vi "GUI_HTT_MultiCamDriveAmpV4.vi"() -> ()   [LabVIEW 2020]
uses:
  Shared/GUI_Template/GUI_master/tcp_new_data_event.ctl
  Shared/GUI_Template/GUI_master/tcp new data cluster.ctl
  General GUIs/Device GUIs/GUI_Cameras/Controls/Crosshair type def.ctl
  <userlib>/_OpenG.lib/array/array.llb/Filter 1D Array with Scalar (String)__ogtk.vi
panel:
  out "Current State":string
  out "String 4":string="x1\ny1\nx2\ny2"
  out "String 3":string="x1\ny1\nx2\ny2"
  out "String 2":string="x1\ny1\nx2\ny2"
  out "String":string="x1\ny1\nx2\ny2"
  in  "visibility":bool=TRUE
  out "appended array":string[](array[string]) caption="XH"
  out "appended array 6":string[](array[string]) caption="XH"
  out "appended array 8":string[](array[string]) caption="XH"
  out "appended array 4":string[](array[string]) caption="XH"
  in  "UDP error message":string
  out "tcp data event 2":T1
  out "error IO 2":errorcluster
  in  "Color Box":u32(colorbox)
  in  "TargetSize.Y::5":dbl=45.0 caption="y" min=2.0 max=3000.0 format="%#_6f"
  in  "TargetSize.X::5":dbl=47.0 caption="x" min=2.0 max=3000.0 format="%#_6f"
  in  "TargetSize.Y::4":dbl=45.0 caption="y" min=2.0 max=3000.0 format="%#_6f"
  in  "TargetSize.X::4":dbl=47.0 caption="x" min=2.0 max=3000.0 format="%#_6f"
  in  "TargetSize.Y::3":dbl=163.0 caption="y" min=2.0 max=3000.0 format="%#_6f"
  in  "TargetSize.X::3":dbl=152.0 caption="x" min=2.0 max=3000.0 format="%#_6f"
  in  "TargetSize.Y::2":dbl=74.0 caption="y" min=2.0 max=3000.0 format="%#_6f"
  in  "TargetSize.X::2":dbl=75.0 caption="x" min=2.0 max=3000.0 format="%#_6f"
  in  "active cams":string
  out "CCDs":string[](array[string])
  out "Cameras":T2
  in  "Target.Y::5":dbl=45.0 caption="y" min=0.0 max=2000.0 format="%#_6f"
  in  "Target.X::5":dbl=47.0 caption="x" min=0.0 max=2000.0 format="%#_6f"
  in  "Target.Y::4":dbl=45.0 caption="y" min=0.0 max=2000.0 format="%#_6f"
  in  "Target.X::4":dbl=47.0 caption="x" min=0.0 max=2000.0 format="%#_6f"
  in  "Target.Y::3":dbl=163.0 caption="y" min=0.0 max=2000.0 format="%#_6f"
  in  "Target.X::3":dbl=152.0 caption="x" min=0.0 max=2000.0 format="%#_6f"
  in  "Target.Y::2":dbl=74.0 caption="y" min=0.0 max=2000.0 format="%#_6f"
  in  "Target.X::2":dbl=75.0 caption="x" min=0.0 max=2000.0 format="%#_6f"
  out "error out":errorcluster
  in  "triggerdelay::5":dbl=0.001 caption="triggerdelay" min=0.0 max=1000000.0 format="%_4p"
  in  "triggerdelay::4":dbl=0.001 caption="triggerdelay" min=0.0 max=1000000.0 format="%_4p"
  in  "triggerdelay::3":dbl=0.001 caption="triggerdelay" min=0.0 max=100000.0 format="%_4p"
  in  "triggerdelay::2":dbl=0.001 caption="triggerdelay" min=0.0 max=1000000.0 format="%_4p"
  in  "trigger::5":bool caption="Trigger"
  in  "centroidy::5":dbl=0.001 caption="centroid y" min=0.0 max=0.0 format="%_4f"
  in  "centroidx::5":dbl=0.001 caption="centroid x" min=0.0 max=0.0 format="%_4f"
  in  "exposure::5":dbl=0.001 caption="exposure" min=9e-05 max=1.0 format="%_4p"
  out "image::5":T3(plugin-control) caption="HTT-MagCam-01"
  in  "GUIdevice 5":string="HTT-D-AMP4_Out"
  in  "trigger::4":bool caption="Trigger"
  in  "centroidy::4":dbl=0.001 caption="centroid y" min=0.0 max=0.0 format="%_4f"
  in  "centroidx::4":dbl=0.001 caption="centroid x" min=0.0 max=0.0 format="%_4f"
  in  "exposure::4":dbl=0.001 caption="exposure" min=9e-05 max=10.0 format="%_4p"
  out "image::4":T3(plugin-control) caption="HTT-MagCam-02"
  in  "GUIdevice 4":string="HTT-D-AMP4_In"
  in  "trigger::3":bool caption="Trigger"
  in  "centroidy::3":dbl=0.001 caption="centroid y" min=0.0 max=0.0 format="%_4f"
  in  "centroidx::3":dbl=0.001 caption="centroid x" min=0.0 max=0.0 format="%_4f"
  in  "exposure::3":dbl=0.001 caption="exposure" min=9e-05 max=10.0 format="%_4p"
  out "image::3":T3(plugin-control) caption="HTT-MagCam-03"
  in  "GUIdevice 3":string="HTT-D-AMP3_In"
  in  "trigger::2":bool caption="Trigger"
  in  "centroidy::2":dbl=0.001 caption="centroid y" min=0.0 max=0.0 format="%_4f"
  in  "centroidx::2":dbl=0.001 caption="centroid x" min=0.0 max=0.0 format="%_4f"
  in  "exposure::2":dbl=0.001 caption="exposure" min=9e-05 max=10.0 format="%_4p"
  out "image::2":T3(plugin-control) caption="HTT-MagCam-04"
  in  "GUIdevice 2":string="HTT-D-AMP2_In"
  out "tcp data event":T1
  in  "Refresh Button":bool caption="Update Crosshairs"
  in  "Select device":string(combo)="FrogHPD"
  in  "stop":bool
  in  "GUIdevice 1":string="HPD_CCD"
  out "image1 4":T3(plugin-control)
  out "image1 3":T3(plugin-control)
  out "image1 2":T3(plugin-control)
  out "image1":T3(plugin-control)
  # "XHair location"
  # "XHair location"
  # "XHair size"
  # "XHair size"
  # "XHair location"
  # "XHair size"
  # "XHair size"
  # "XHair location"
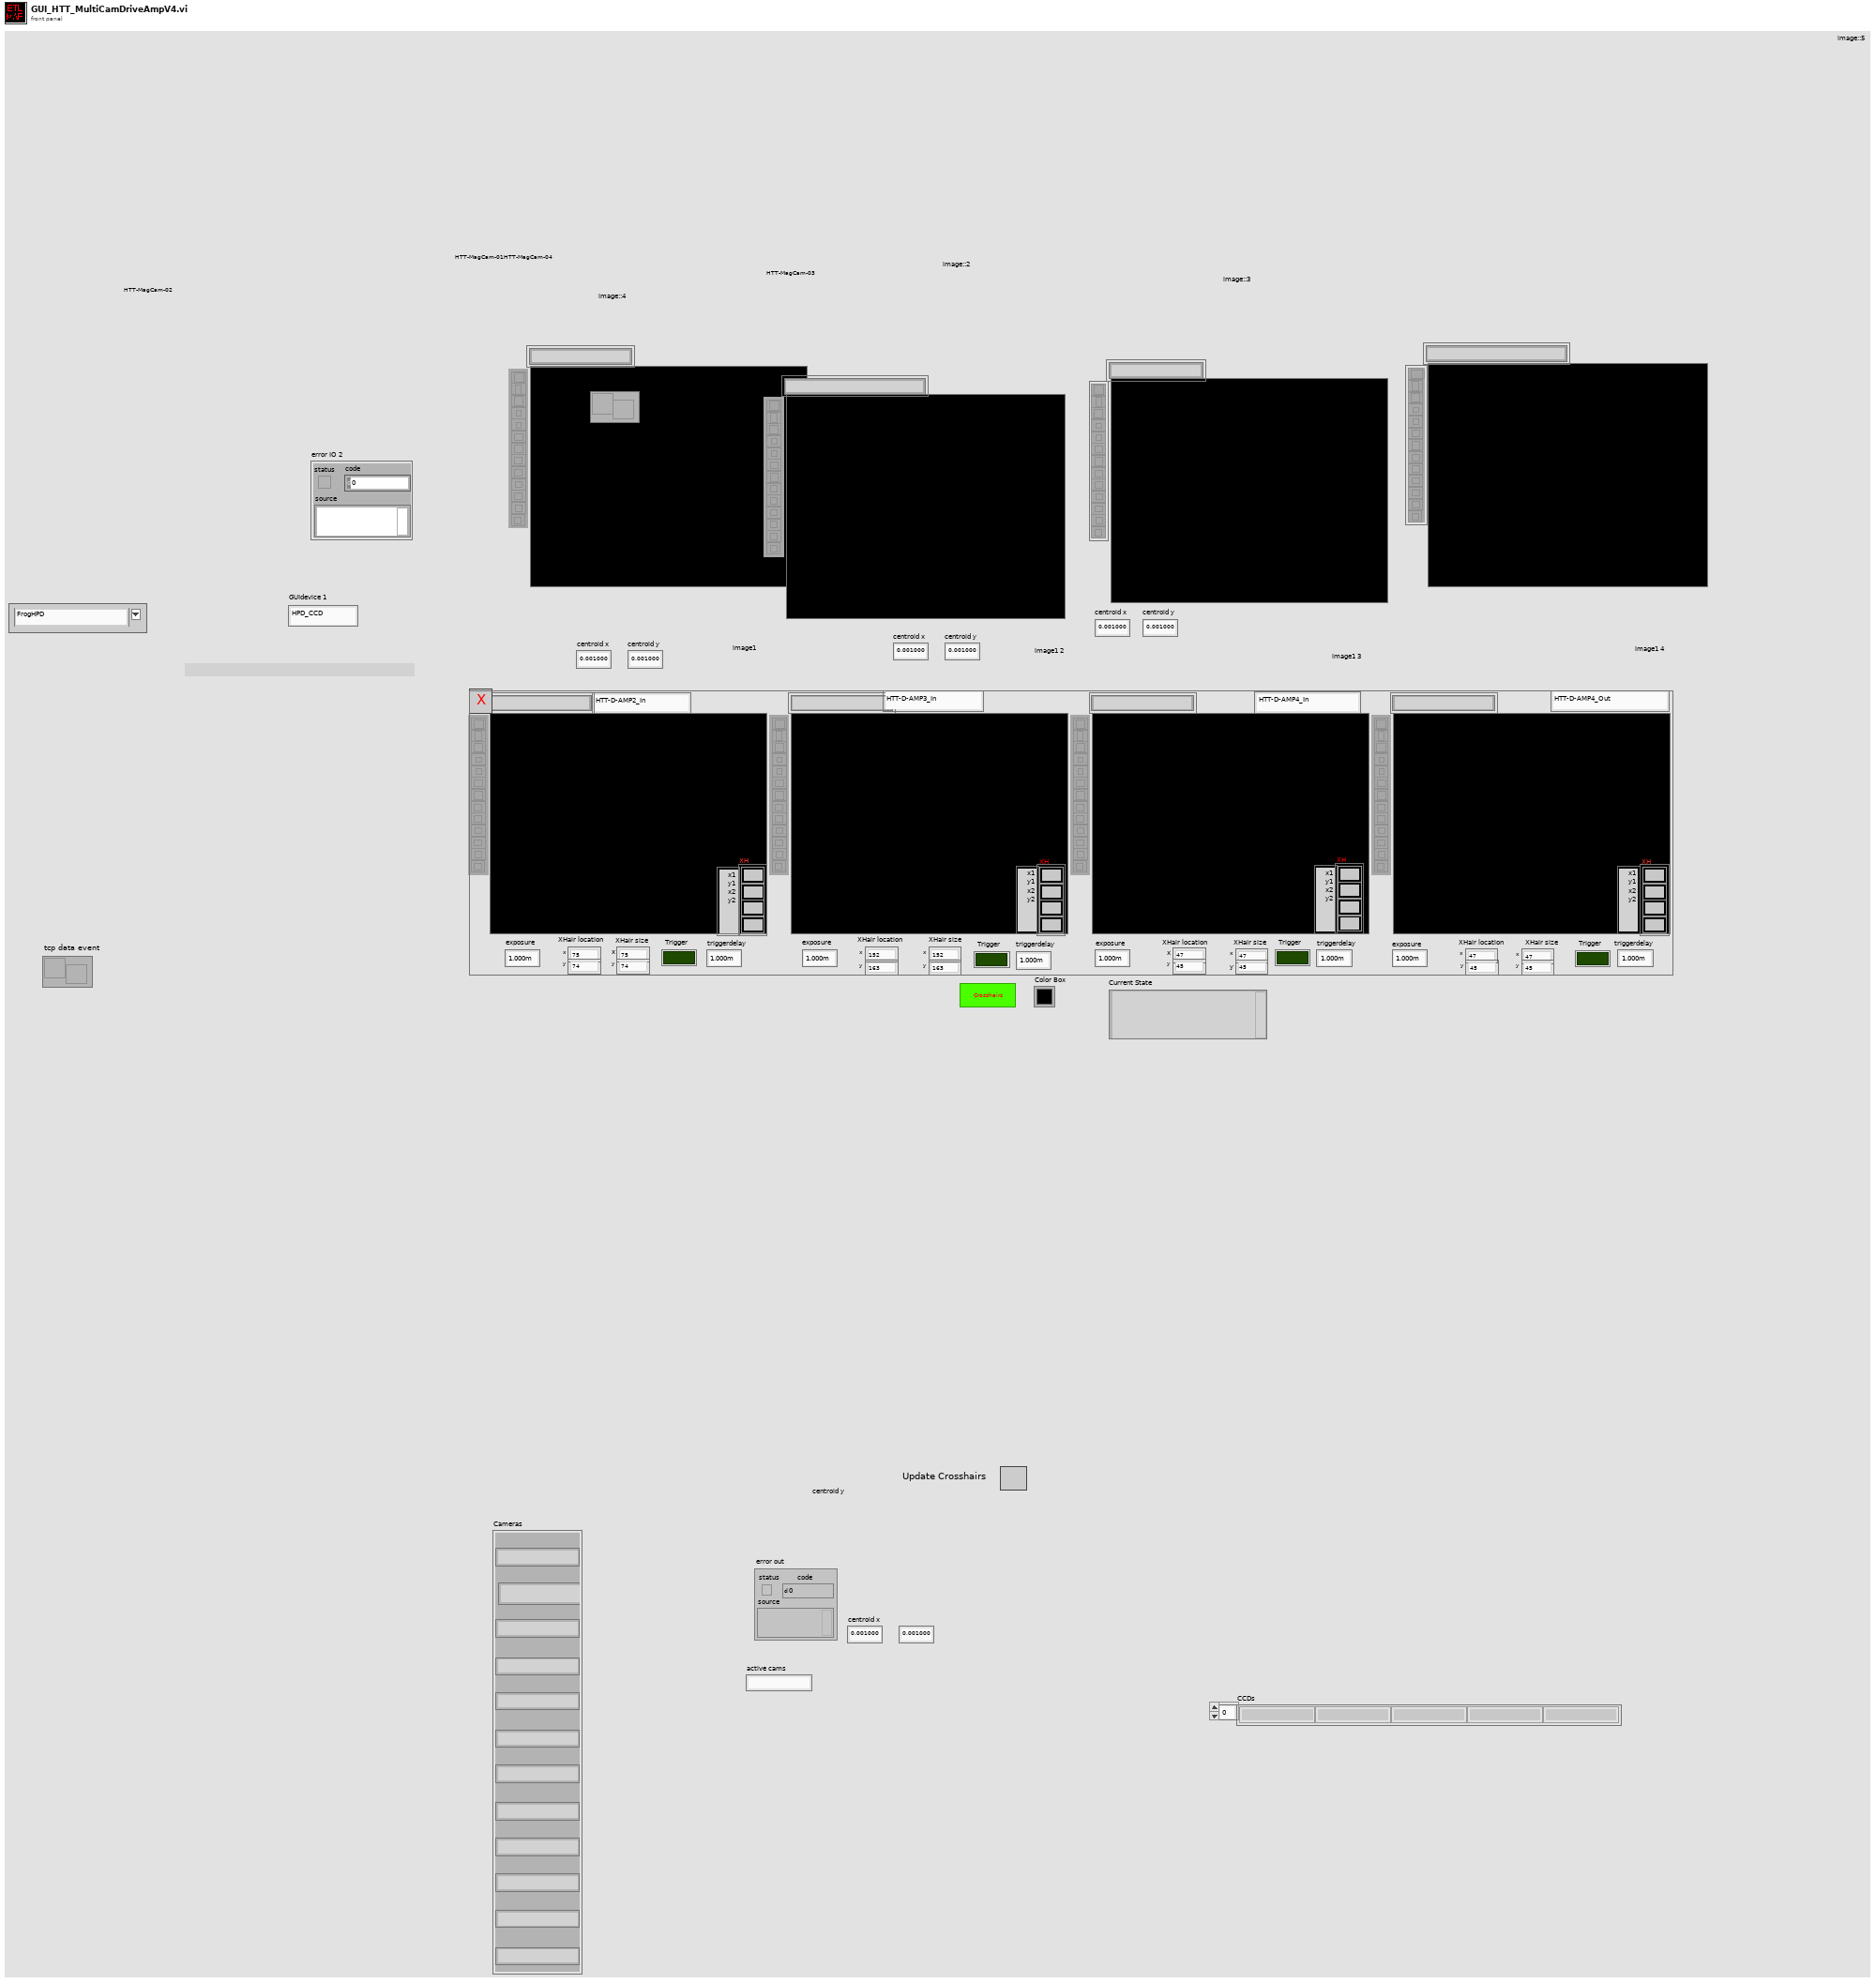
[diagram p1: front panel]
types:
  T1 = typedef "tcp_new_data_event.ctl" = refnum<user-event>
  T2 = cluster{"[0]":string, "[1]":string, "[2]":string, "[3]":string, "[4]":string, "[5]":string, "[6]":string, "[7]":string, "[8]":string, "[8] 2":string, "[8] 3":string, "[8] 4":string}
  T3 = typedef "IMAQ Image.ctl" = refnum<image>
  T4 = typedef "Image Type" = u32
  T5 = cluster{"Target.X::2":refnum<vi>, "Target.Y::2":refnum<vi>}
  T6 = cluster{"Target.X::3":refnum<vi>, "Target.Y::3":refnum<vi>}
  T7 = cluster{"Target.X::4":refnum<vi>, "Target.Y::4":refnum<vi>}
  T8 = cluster{"Target.X::5":refnum<vi>, "Target.Y::5":refnum<vi>}
  T9 = cluster{"TargetSize.X::2":refnum<vi>, "TargetSize.Y::2":refnum<vi>}
  T10 = cluster{"TargetSize.X::3":refnum<vi>, "TargetSize.Y::3":refnum<vi>}
  T11 = cluster{"TargetSize.X::4":refnum<vi>, "TargetSize.Y::4":refnum<vi>}
  T12 = cluster{"TargetSize.X::5":refnum<vi>, "TargetSize.Y::5":refnum<vi>}
  T13 = cluster{"Target.X::5":refnum<vi>, "Target.Y::5":refnum<vi>}[]
  T14 = cluster{"TargetSize.X::5":refnum<vi>, "TargetSize.Y::5":refnum<vi>}[]
  T15 = cluster{"[0]":string, "[1]":string, "[2]":string, "[3]":string, "[4]":string, "[5]":string, "[6]":string, "[7]":string, "[8]":string, "[9]":string, "[10]":string, "[11]":string}
  T16 = typedef "Crosshair type def.ctl" = cluster{"Draw":bool, "Target":cluster{"x":dbl, "y":dbl}, "Size":cluster{"x":dbl, "y":dbl}, "Angle":dbl, "Color":u32, "Thickness":u8, "CrosshairLabel":string}
  T17 = cluster{"Left":i32, "Top":i32, "Right":i32, "Bottom":i32}
  T18 = enum32{"invalid app kind", "Development System", "Run Time System", "Student Edition", "Embedded LabVIEW", "Evaluation", "Custom"}
  T19 = typedef "tcp new data cluster.ctl" = cluster{"EventEnum":enum16{"new data", "connection status update"}, "Device name":string}
  T20 = enum32{"Invalid", "Standard", "Closed", "Hidden", "Minimized", "Maximized"}
  T21 = cluster{"Core":cluster{"Current VI Reference":refnum<vi>, "Close Panel on Exit?":bool}, "Your Boolean data":bool, "active cams":string, "SuperGUI":cluster{"STOP queue":refnum<queue>, "SuperGUI ref":refnum<vi>}}
  T22 = cluster{"STOP queue":refnum<queue>, "SuperGUI ref":refnum<vi>}
  T23 = cluster{"Current VI Reference":refnum<vi>, "Close Panel on Exit?":bool}
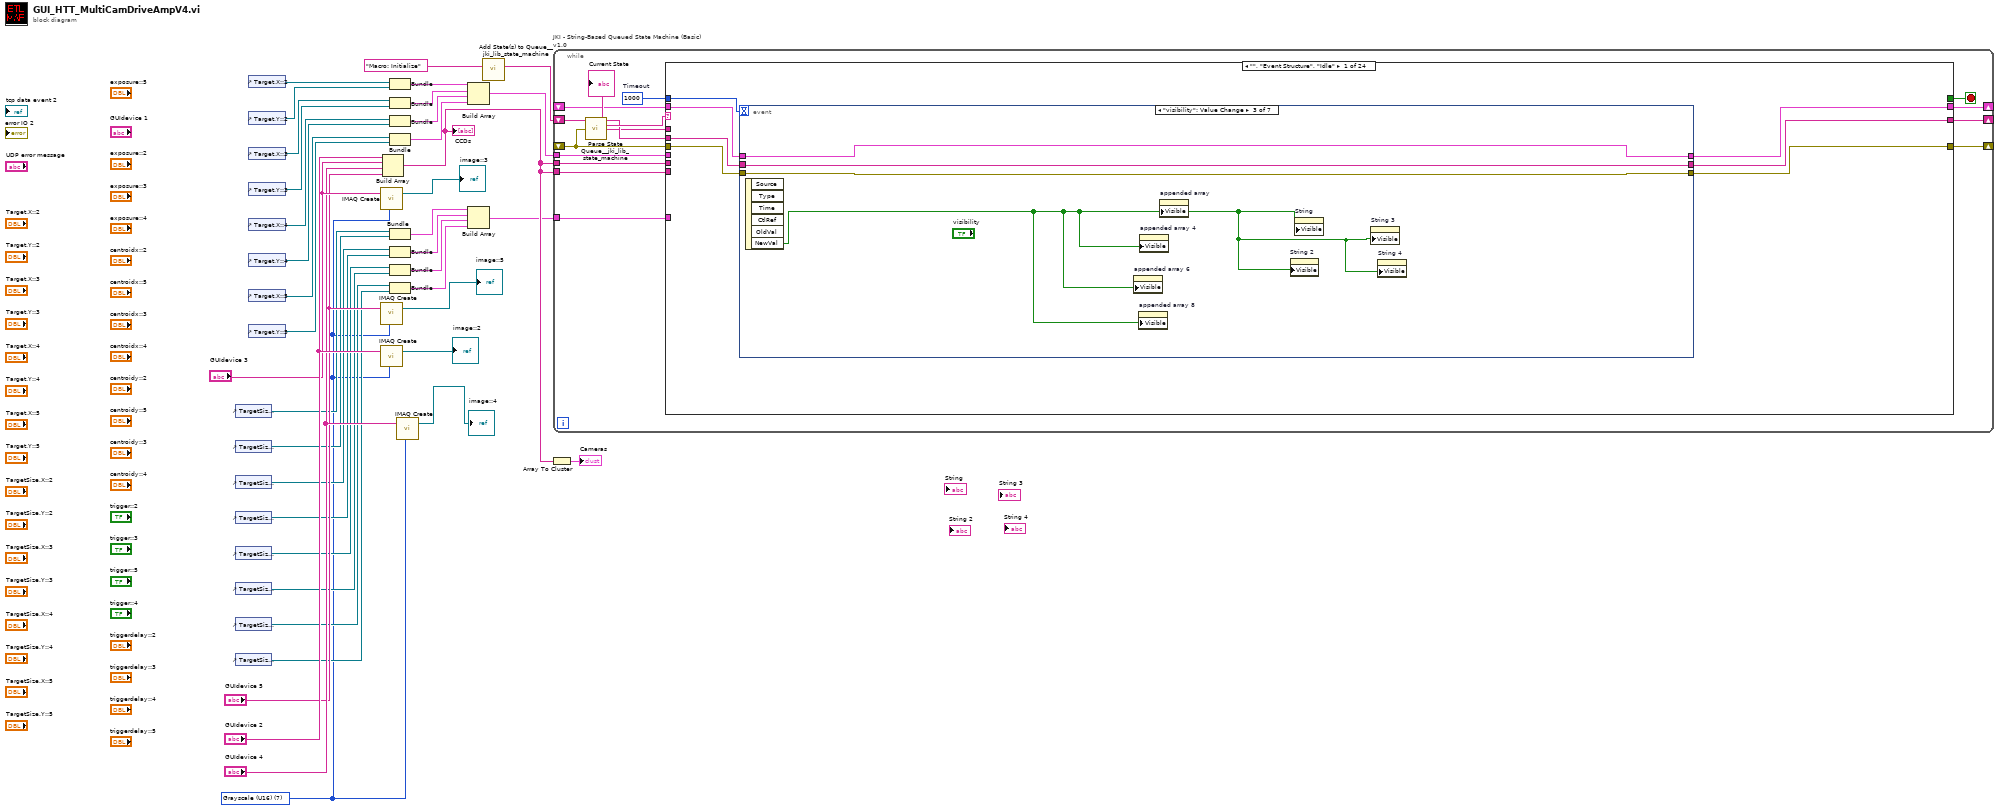
[diagram p0: block diagram]
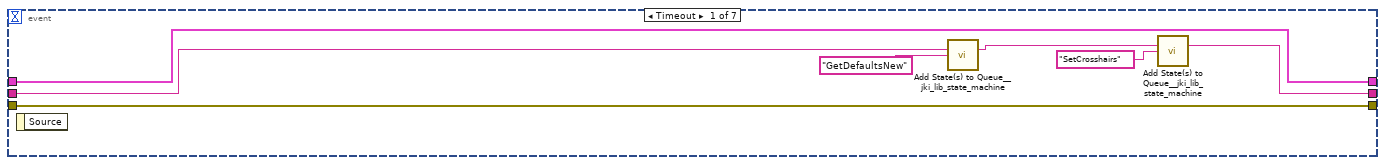
[diagram p2: hidden frame]
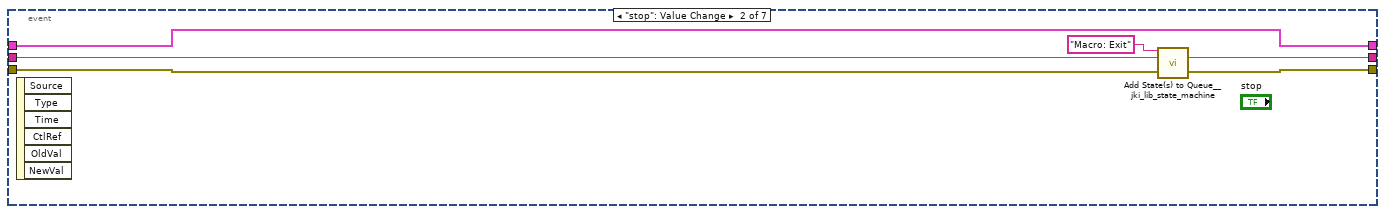
[diagram p3: hidden frame]
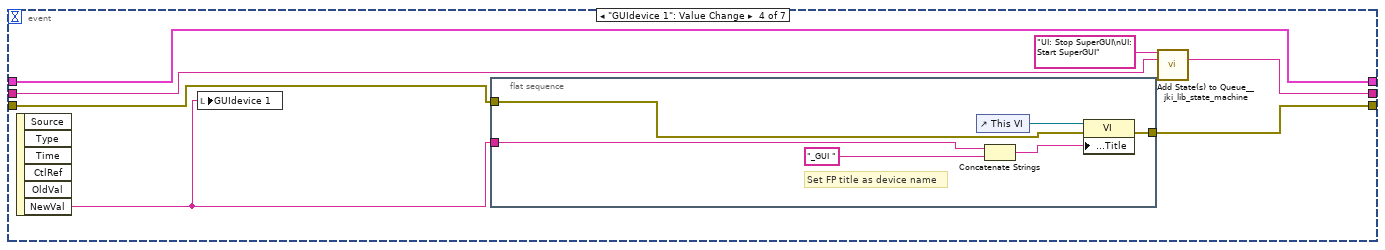
[diagram p4: hidden frame]
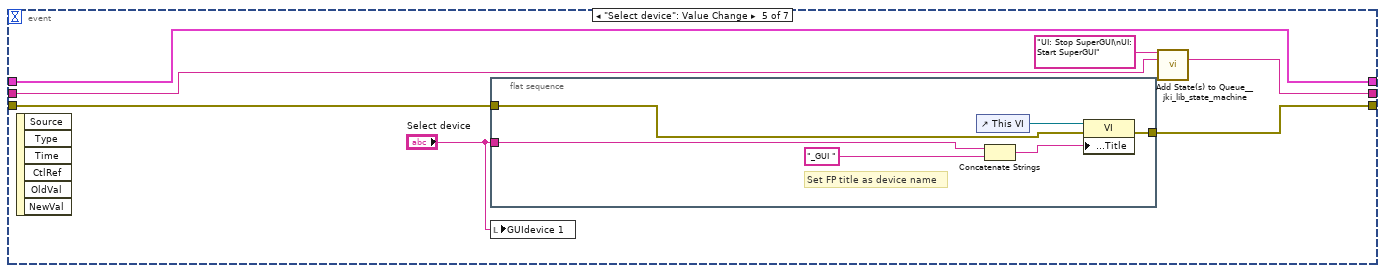
[diagram p5: hidden frame]
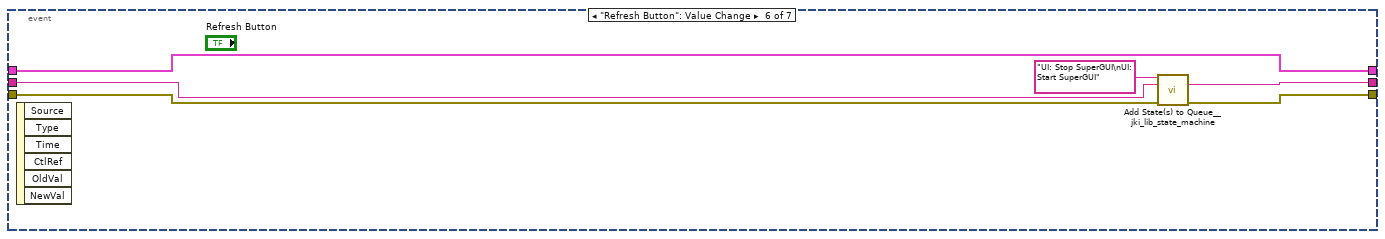
[diagram p6: hidden frame]
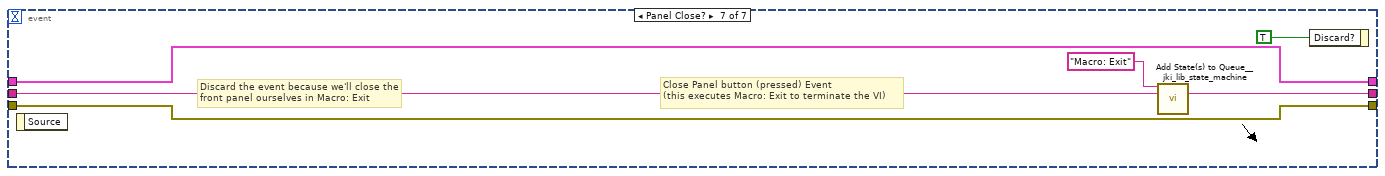
[diagram p7: hidden frame]
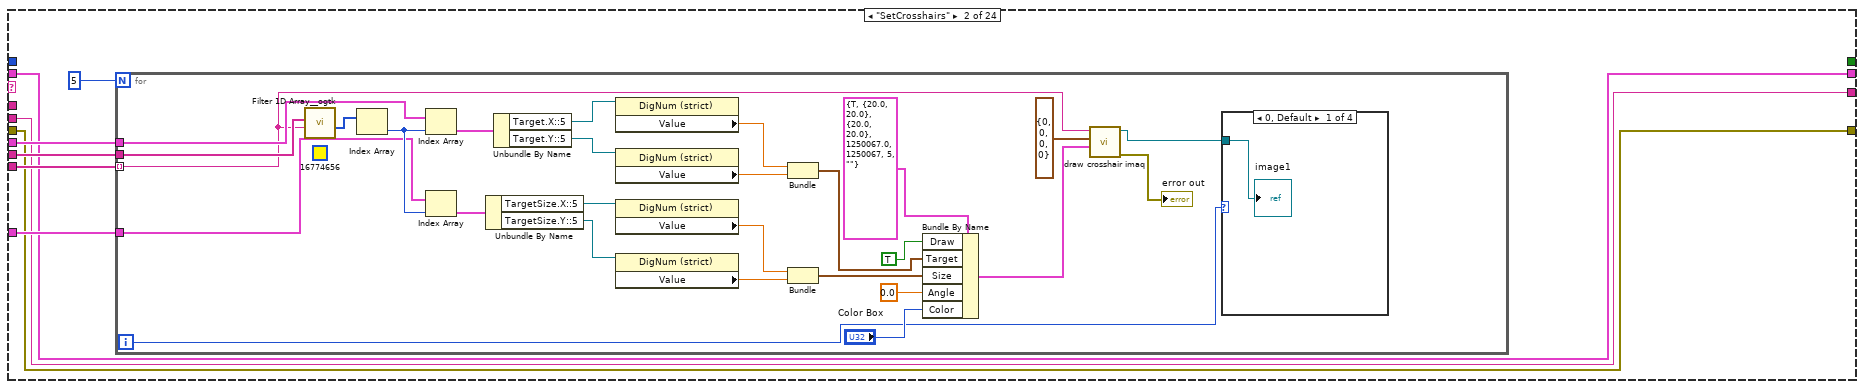
[diagram p8: hidden frame]
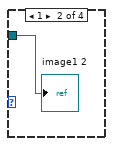
[diagram p9: hidden frame]
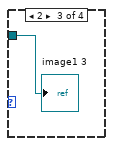
[diagram p10: hidden frame]
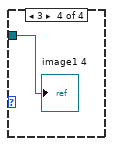
[diagram p11: hidden frame]
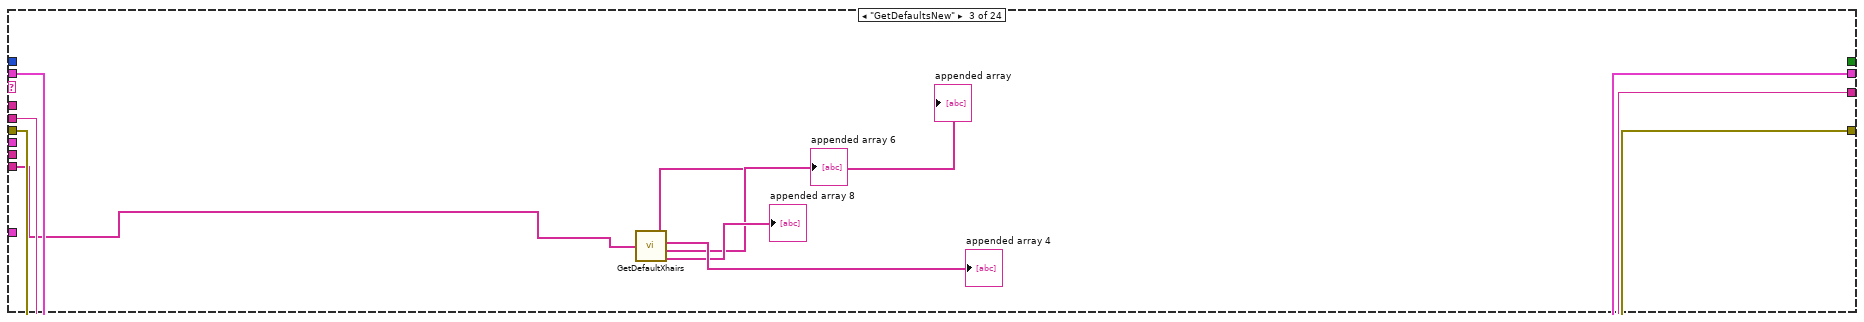
[diagram p12: hidden frame]
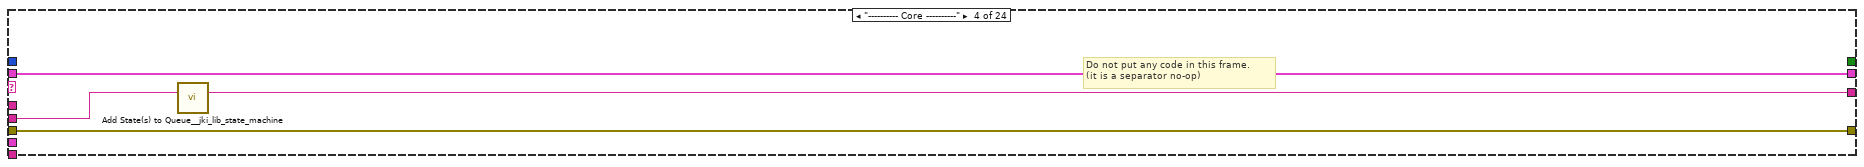
[diagram p13: hidden frame]
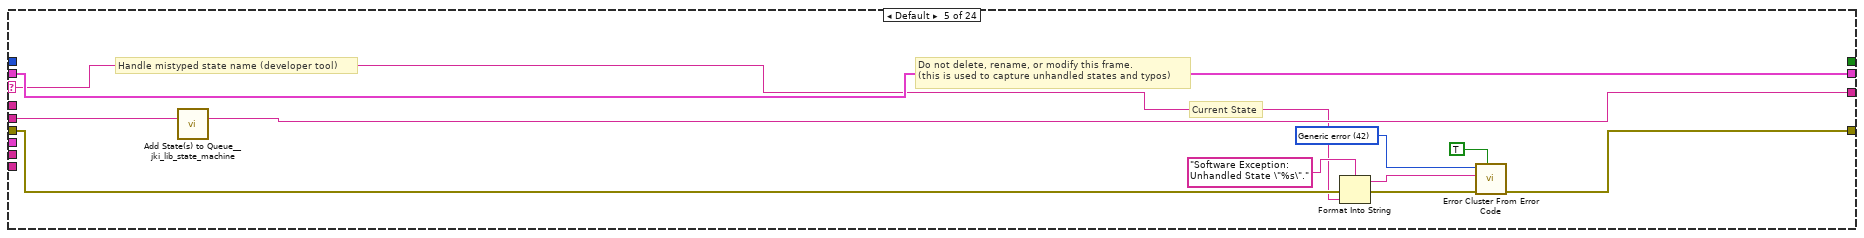
[diagram p14: hidden frame]
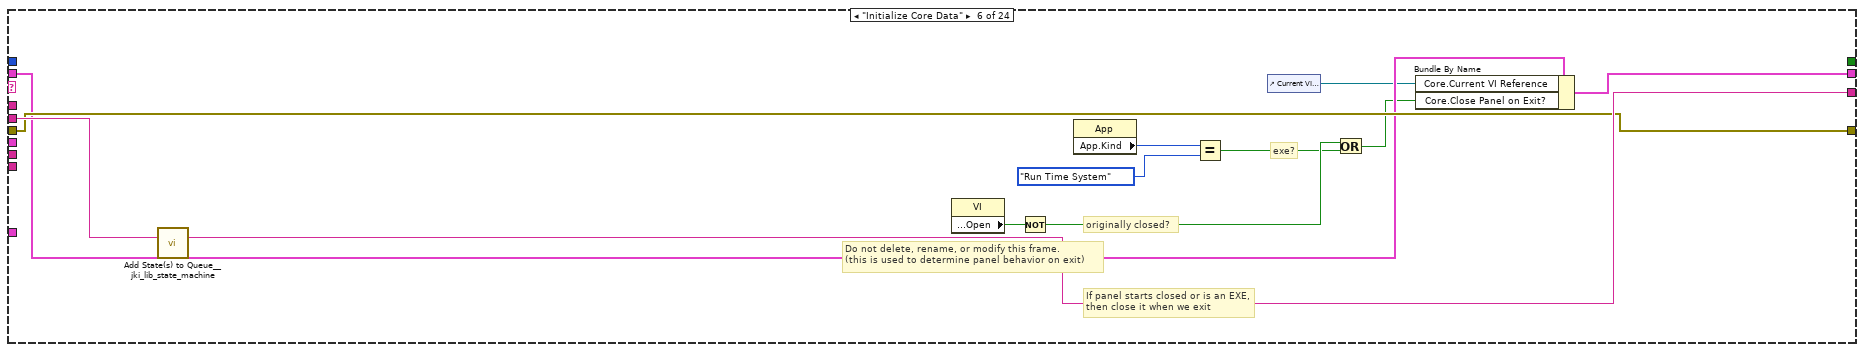
[diagram p15: hidden frame]
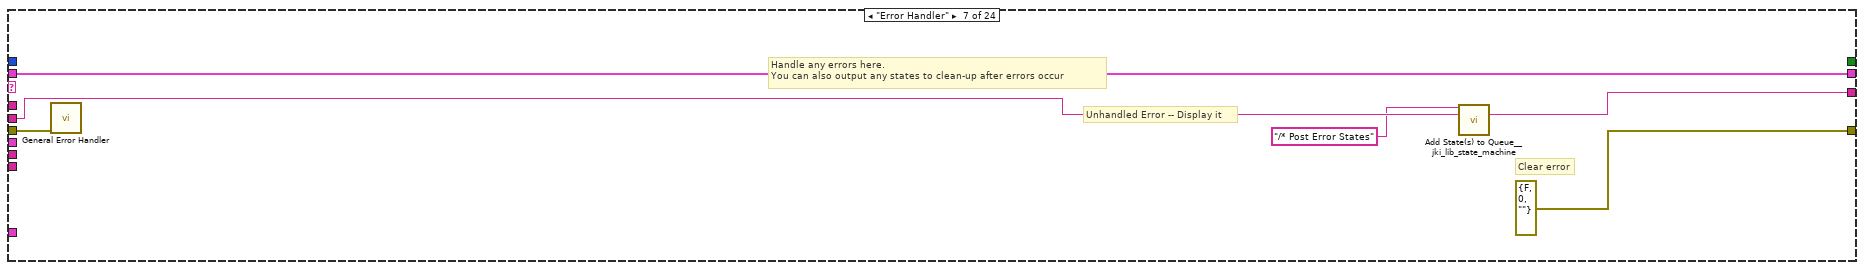
[diagram p16: hidden frame]
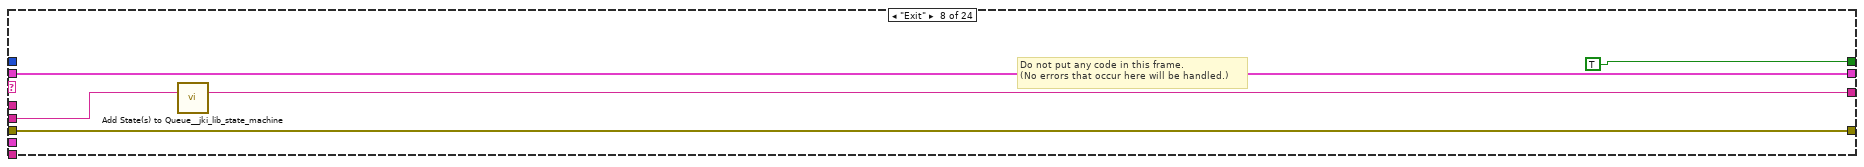
[diagram p17: hidden frame]
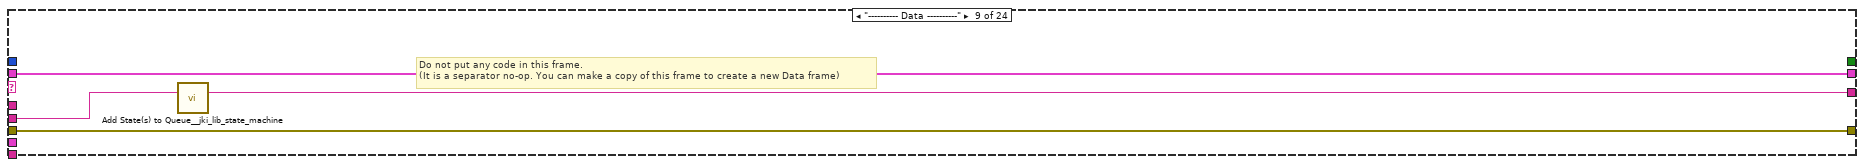
[diagram p18: hidden frame]
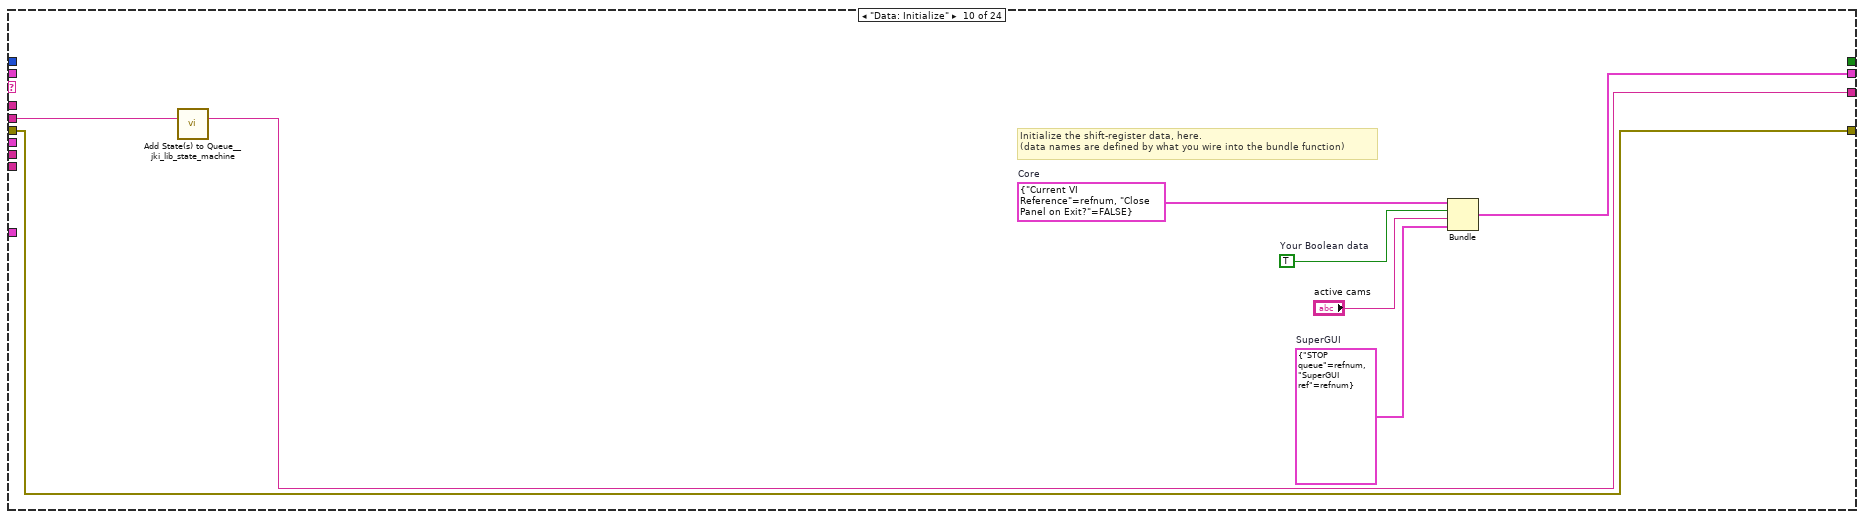
[diagram p19: hidden frame]
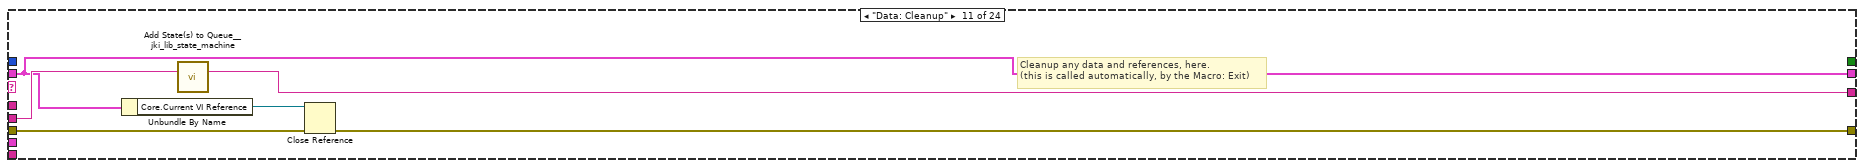
[diagram p20: hidden frame]
diagram:
  w2 = T4 7 items=["Grayscale (U8)", "Grayscale (I16)", "Grayscale (SGL)", "Complex (CSG)", "RGB (U32)", "HSL (U32)", "RGB (U64)", "Grayscale (U16)"] ("Image Type")
  n1 = control-ref of="TargetSize.X::2"() -> (w15:refnum<vi>)
  n2 = control-ref of="TargetSize.Y::2"() -> (w14:refnum<vi>)
  n3 = control-ref of="TargetSize.X::3"() -> (w13:refnum<vi>)
  n4 = control-ref of="TargetSize.Y::3"() -> (w12:refnum<vi>)
  n5 = control-ref of="TargetSize.X::4"() -> (w11:refnum<vi>)
  n6 = control-ref of="TargetSize.Y::4"() -> (w10:refnum<vi>)
  n7 = control-ref of="TargetSize.X::5"() -> (w9:refnum<vi>)
  n8 = control-ref of="TargetSize.Y::5"() -> (w8:refnum<vi>)
  n9 = control-ref of="Target.X::2"() -> (w34:refnum<vi>)
  n10 = control-ref of="Target.Y::2"() -> (w33:refnum<vi>)
  n11 = control-ref of="Target.X::3"() -> (w32:refnum<vi>)
  n12 = control-ref of="Target.Y::3"() -> (w31:refnum<vi>)
  n13 = control-ref of="Target.X::4"() -> (w30:refnum<vi>)
  n14 = control-ref of="Target.Y::4"() -> (w29:refnum<vi>)
  n15 = control-ref of="Target.X::5"() -> (w28:refnum<vi>)
  n16 = control-ref of="Target.Y::5"() -> (w27:refnum<vi>)
  n17 = call "IMAQ Create"("Image Name"="GUIdevice 3", "Image Type"=w2) -> ("New Image"=→"image::3":T3)  [unwired: 3 in, 1 out]
  n18 = call "IMAQ Create"("Image Name"="GUIdevice 5", "Image Type"=w2) -> ("New Image"=→"image::5":T3)  [unwired: 3 in, 1 out]
  n19 = call "IMAQ Create"("Image Name"="GUIdevice 2", "Image Type"=w2) -> ("New Image"=→"image::2":T3)  [unwired: 3 in, 1 out]
  n20 = Build Array("GUIdevice 2", "GUIdevice 3", "GUIdevice 4", "GUIdevice 5") -> (w16:string[])
  "CCDs" <- w16
  n21 = Bundle("Target.X::2"=w34, "Target.Y::2"=w33) -> (w26:T5)  [unwired: 1 in]
  n22 = Bundle("Target.X::3"=w32, "Target.Y::3"=w31) -> (w25:T6)  [unwired: 1 in]
  n23 = Bundle("Target.X::4"=w30, "Target.Y::4"=w29) -> (w23:T7)  [unwired: 1 in]
  n24 = Bundle("Target.X::5"=w28, "Target.Y::5"=w27) -> (w24:T8)  [unwired: 1 in]
  n25 = Bundle("TargetSize.X::2"=w15, "TargetSize.Y::2"=w14) -> (w7:T9)  [unwired: 1 in]
  n26 = Bundle("TargetSize.X::3"=w13, "TargetSize.Y::3"=w12) -> (w6:T10)  [unwired: 1 in]
  n27 = Bundle("TargetSize.X::4"=w11, "TargetSize.Y::4"=w10) -> (w4:T11)  [unwired: 1 in]
  n28 = Bundle("TargetSize.X::5"=w9, "TargetSize.Y::5"=w8) -> (w5:T12)  [unwired: 1 in]
  n29 = call "IMAQ Create"("Image Name"="GUIdevice 4", "Image Type"=w2) -> ("New Image"=→"image::4":T3)  [unwired: 3 in, 1 out]
  n30 = Build Array(w26, w25, w23, w24) -> (w22:T13)
  n31 = Build Array(w7, w6, w4, w5) -> (w3:T14)
  n32 = call <vilib>:"Add State(s) to Queue__jki_lib_state_machine.vi"("State(s) in (\"\")"="Macro: Initialize") -> ("States Out"=w39:string)  [unwired: 14 in]
  n33 = Array To Cluster(array=w16) -> (cluster=→"Cameras":T15)
  n34 = while "JKI - String-Based Queued State Machine (Basic) v1.0" {
    shift-right: [w47] -> _
    shift-left: _ -> [w44]
    shift-right: [w50] -> _
    shift-left: _ -> [w45]
    shift-right: [w49] -> _
    shift-left: w39 -> [w51]
    tunnel: w22 -> [w41]
    tunnel: w16 -> [w42]
    tunnel: w16 -> [w43]
    tunnel: w3 -> [w40]
    stop <- w48 stop-if-true
    w46 = 1000  # Timeout
    n35 = call <vilib>:"Parse State Queue__jki_lib_state_machine.vi"("State Queue"=w51, "Error In (no error)"=w45) -> ("Remaining States"=w53:string, "Current State"=w54:string, "Arguments"=w52:string)  [unwired: 11 in]
    "Current State" <- w54
    n36 = case shown="\"\", \"Event Structure\", \"Idle\"" w54 {
      selector: w54 -> [_ _ _ _ w166 _ _ _ _ _ _ _ _ _ _ _ _ _ _ _ _ _ _ _]
      tunnel: w53 -> [w61 w117 w160 w165 w170 w188 w194 w199 w203 w211 w217 w221 w226 w232 w267 w275 w281 w292 w318 w323 w334 w338 w342 w346]
      tunnel: w52 -> [_ _ _ _ _ _ _ _ _ _ _ _ _ _ _ _ w276 w286 _ _ _ _ _ _]
      tunnel: w44 -> [w59 w118 w161 w162 w168 w179 w191 w197 w200 _ w212 w218 w224 w230 w258 w270 w279 w288 w315 w320 w331 w335 w339 w343]
      tunnel: [w58 w116 w159 w163 w172 w185 errorcluster {"status"=FALSE, "code"=0, "source"=""} ("error out") w196 w201 w208 w213 w219 w222 w227 w251 w268 w277 w289 w316 w321 w332 w336 w340 w344] -> w50
      tunnel: w45 -> [w57 w116 w159 w163 w171 w185 w190 w196 w201 w208 w214 w219 w223 w228 w252 w269 w278 w290 w316 w321 w332 w336 w340 w344]
      tunnel: [w60 w117 w160 w164 w169 w187 w193 w198 w202 w210 w216 w220 w225 w231 w266 w274 w280 w291 w317 w322 w333 w337 w341 w345] -> w49
      tunnel: [_ _ _ _ _ _ _ TRUE _ _ _ _ _ _ _ _ _ _ _ _ _ _ _ _] -> w48
      tunnel: [w56 w118 w161 w162 w168 w186 w191 w197 w200 w209 w212 w218 w224 w230 w257 w270 w279 w288 w315 w320 w331 w335 w339 w343] -> w47
      tunnel: w46 -> [w55 _ _ _ _ _ _ _ _ _ _ _ _ _ _ _ _ _ _ _ _ _ _ _]
      tunnel: w43 -> [_ w120 w158 _ _ _ _ _ _ _ _ _ _ _ _ _ _ _ _ _ _ _ _ _]
      tunnel: w42 -> [_ w121 _ _ _ _ _ _ _ _ _ _ _ _ _ _ _ _ _ _ _ _ _ _]
      tunnel: w41 -> [_ w122 _ _ _ _ _ _ _ _ _ _ _ _ _ _ _ _ _ _ _ _ _ _]
      tunnel: w40 -> [_ w119 _ _ _ _ _ _ _ _ _ _ _ _ _ _ _ _ _ _ _ _ _ _]
      frame "", "Event Structure", "Idle" {
        n37 = event shown="[2] \"visibility\": Value Change" {
          selector: _ -> [_ _ _ _ _ _ _]
          dyn-events: _ -> [_ _ _ _ _ _ _]
          timeout: w55 -> [_ _ _ _ _ _ _]
          tunnel: w61 -> [w64 w71 w75 w81 w93 w106 w114]
          tunnel: [w68 w70 w75 w80 w92 w105 w113] -> w60
          tunnel: w59 -> [w66 w73 w77 w84 w97 w108 w111]
          tunnel: [w67 w72 w76 w82 w95 w107 w112] -> w58
          tunnel: w57 -> [w67 w72 w76 w83 w96 w107 w112]
          tunnel: [w66 w73 w77 w84 w97 w108 w111] -> w56
          event Timeout {
            n38 = event-data() -> ()  [unwired: 1 in, 1 out]
            n39 = call <vilib>:"Add State(s) to Queue__jki_lib_state_machine.vi"("State(s) in (\"\")"=w64, "State(s) at Back (\"\")"="GetDefaultsNew") -> ("States Out"=w62:string)  [unwired: 13 in]
            n40 = call <vilib>:"Add State(s) to Queue__jki_lib_state_machine.vi"("State(s) in (\"\")"=w62, "State(s) at Back (\"\")"="SetCrosshairs") -> ("States Out"=w68:string)  [unwired: 13 in]
          }
          event "stop": Value Change {
            n41 = event-data() -> ()  [unwired: 1 in, 6 out]
            n42 = call <vilib>:"Add State(s) to Queue__jki_lib_state_machine.vi"("State(s) in Front (\"\")"="Macro: Exit", "State(s) in (\"\")"=w71) -> ("States Out"=w70:string)  [unwired: 13 in]
          }
          event "visibility": Value Change {
            n43 = event-data() -> ("NewVal"=w74:bool)  [unwired: 1 in, 5 out]
            n44 = property on="appended array 6" class="Arr (strict)"("Visible"=w74) -> ()  [unwired: 2 in, 2 out]
            n45 = property on="appended array 8" class="Arr (strict)"("Visible"=w74) -> ()  [unwired: 2 in, 2 out]
            n46 = property on="appended array 4" class="Arr (strict)"("Visible"=w74) -> ()  [unwired: 2 in, 2 out]
            n47 = property on="appended array" class="Arr (strict)"("Visible"=w74) -> ()  [unwired: 2 in, 2 out]
            n48 = property on="String 2" class="Str"("Visible"=w74) -> ()  [unwired: 2 in, 2 out]
            n49 = property on="String" class="Str"("Visible"=w74) -> ()  [unwired: 2 in, 2 out]
            n50 = property on="String 3" class="Str"("Visible"=w74) -> ()  [unwired: 2 in, 2 out]
            n51 = property on="String 4" class="Str"("Visible"=w74) -> ()  [unwired: 2 in, 2 out]
          }
          event "GUIdevice 1": Value Change {
            n52 = event-data() -> ("NewVal"=w78:string)  [unwired: 1 in, 5 out]
            n53 = local write "GUIdevice 1"(w78) -> ()
            n54 = flat-sequence {
              tunnel: [w87] -> w82
              tunnel: w83 -> [w86]
              tunnel: w78 -> [w85]
              frame #0 {
                # "Set FP title as device name"
                n55 = control-ref of="This VI"() -> (w90:refnum<vi>)
                n56 = Concatenate Strings(w85, "_GUI ") -> (w89:string)
                n57 = property class="VI"(reference=w90, error in=w86, "Front Panel.Title"=w89) -> (error out=w87:errorcluster)  [unwired: 1 out]
              }
            }
            n58 = call <vilib>:"Add State(s) to Queue__jki_lib_state_machine.vi"("State(s) in Front (\"\")"="UI: Stop SuperGUI\nUI: Start SuperGUI", "State(s) in (\"\")"=w81) -> ("States Out"=w80:string)  [unwired: 13 in]
          }
          event "Select device": Value Change {
            n59 = event-data() -> ()  [unwired: 1 in, 6 out]
            n60 = flat-sequence {
              tunnel: [w100] -> w95
              tunnel: w96 -> [w99]
              tunnel: "Select device" -> [w98]
              frame #0 {
                # "Set FP title as device name"
                n61 = control-ref of="This VI"() -> (w103:refnum<vi>)
                n62 = Concatenate Strings(w98, "_GUI ") -> (w102:string)
                n63 = property class="VI"(reference=w103, error in=w99, "Front Panel.Title"=w102) -> (error out=w100:errorcluster)  [unwired: 1 out]
              }
            }
            n64 = local write "GUIdevice 1"("Select device") -> ()
            n65 = call <vilib>:"Add State(s) to Queue__jki_lib_state_machine.vi"("State(s) in Front (\"\")"="UI: Stop SuperGUI\nUI: Start SuperGUI", "State(s) in (\"\")"=w93) -> ("States Out"=w92:string)  [unwired: 13 in]
          }
          event "Refresh Button": Value Change {
            n66 = event-data() -> ()  [unwired: 1 in, 6 out]
            n67 = call <vilib>:"Add State(s) to Queue__jki_lib_state_machine.vi"("State(s) in Front (\"\")"="UI: Stop SuperGUI\nUI: Start SuperGUI", "State(s) in (\"\")"=w106) -> ("States Out"=w105:string)  [unwired: 13 in]
          }
          event Panel Close? {
            # "Discard the event because we'll close the front panel ourselves in Macro: Exit"
            # "Close Panel button (pressed) Event\n(this executes Macro: Exit to terminate the VI)"
            n68 = event-data() -> ()  [unwired: 1 in, 1 out]
            n69 = call <vilib>:"Add State(s) to Queue__jki_lib_state_machine.vi"("State(s) in Front (\"\")"="Macro: Exit", "State(s) in (\"\")"=w114) -> ("States Out"=w113:string)  [unwired: 13 in]
            n70 = event-data("Discard?"=TRUE) -> ()  [unwired: 1 in, 1 out]
          }
        }
      }
      frame "SetCrosshairs" {
        n71 = for {
          N: 5 -> [_]
          tunnel: w121 -> [w128]
          tunnel: w122 -> [w127]
          tunnel: w119 -> [w126]
          tunnel: w120 -> [w125] mode=indexing
          i -> [w124]
          (unwired) u32 16774656 ("Color")
          n72 = call-poly <userlib>:"Filter 1D Array__ogtk.vi"("items to filter"=w125, "array"=w128) -> ("filtered item indices"=w132:i32[])  [unwired: 4 in, 1 out]
          n73 = Index Array(array=w132) -> (element=w135:i32)  [unwired: 1 in]
          n74 = Index Array(array=w127, index=w135) -> (element=w133:T8)
          n75 = Index Array(array=w126, index=w135) -> (element=w136:T12)
          n76 = Unbundle By Name(w136) -> ("TargetSize.X::5"=w137:refnum<vi>, "TargetSize.Y::5"=w138:refnum<vi>)
          n77 = Unbundle By Name(w133) -> ("Target.X::5"=w130:refnum<vi>, "Target.Y::5"=w131:refnum<vi>)
          n78 = property class="DigNum (strict)"(reference=w130) -> ("Value"=w144:dbl)  [unwired: 1 in, 2 out]
          n79 = property class="DigNum (strict)"(reference=w131) -> ("Value"=w145:dbl)  [unwired: 1 in, 2 out]
          n80 = property class="DigNum (strict)"(reference=w137) -> ("Value"=w139:dbl)  [unwired: 1 in, 2 out]
          n81 = property class="DigNum (strict)"(reference=w138) -> ("Value"=w140:dbl)  [unwired: 1 in, 2 out]
          n82 = Bundle("Value"=w144, "Value"=w145) -> (w146:cluster{"Value":dbl, "Value":dbl})  [unwired: 1 in]
          n83 = Bundle("Value"=w139, "Value"=w140) -> (w147:cluster{"Value":dbl, "Value":dbl})  [unwired: 1 in]
          n84 = Bundle By Name(cluster=T16 {"Draw"=TRUE, "Target"={"x"=20.0, "y"=20.0}, "Size"={"x"=20.0, "y"=20.0}, "Angle"=1250067.0, "Color"=1250067, "Thickness"=5, "CrosshairLabel"=""} ("Crosshair"), "Draw"=TRUE, "Target"=w146, "Size"=w147, "Angle"=0.0, "Color"="Color Box") -> (w142:T16)
          n85 = call "draw crosshair imaq.vi"("Crosshair"=w142, "Bounding Rectangle"=T17 {"Left"=0, "Top"=0, "Right"=0, "Bottom"=0}, "image in"=w125) -> ("error out"=→"error out":errorcluster, "image out"=w123:T3)  [unwired: 7 in]
          n86 = case shown="0, Default" w124 {
            tunnel: w123 -> [w150 w151 w152 w153]
            frame 0, Default {
              "image1" <- w150
            }
            frame 1 {
              "image1 2" <- w151
            }
            frame 2 {
              "image1 3" <- w152
            }
            frame 3 {
              "image1 4" <- w153
            }
          }
        }
      }
      frame "GetDefaultsNew" {
        n87 = call "GetDefaultXhairs.vi"("appended array 2"=w158) -> ("appended array"=→"appended array":string[], "appended array 4"=→"appended array 4":string[], "appended array 6"=→"appended array 6":string[], "appended array 8"=→"appended array 8":string[])
      }
      frame "---------- Core ----------" {
        # "Do not put any code in this frame.\n(it is a separator no-op)"
        n88 = call <vilib>:"Add State(s) to Queue__jki_lib_state_machine.vi"("State(s) in (\"\")"=w165) -> ("States Out"=w164:string)  [unwired: 14 in]
      }
      frame Default {
        w175 = 42 items=["No error", "Argument error", "Memory is full", "Out of zone", "End of file", "File already open", "Generic file I/O error", "File not found", "File permission error", "Disk is full", "Duplicate path", "Too many files open", "System feature not enabled", "Resource file not found", "Cannot add resource", "Resource not found", "Image not found", "Image memory error", "Pen does not exist", "Config type invalid", "Config token not found", "Config parse error", "Config memory error", "Bad external code format", "Bad external code offset", "External code not present", "Null window", "Destroy window error", "Null menu", "Print aborted", "Bad print record", "Print driver error", "Windows error during printing", "Memory error during printing", "Print dialog error", "Generic print error", "Invalid device refnum", "Device not found", "Device parameter error", "Device unit error", "Cannot open device", "Device call aborted", "Generic error", "Cancelled by user", "Object ID too low", "Object ID too high", "Object not in heap", "Unknown heap", "Unknown object (invalid DefProc)", "Unknown object (DefProc not in table)", "Message out of range", "Invalid (null) method", "Unknown message", "Manager call not supported", "Bad address", "Network operation in progress", "Network operation timed out", "Connection is busy", "Network attribute not supported", "Network error", "Address in use", "System out of memory", "Connection aborted", "Connection refused", "Not connected", "Already connected", "Connection closed", "Initialization error (interapplication manager)", "Bad occurrence", "Wait on unbound occurrence handler", "Occurrence queue overflow", "Datalog type conflict", "Unused", "Unrecognized type (interapplication manager)", "Memory corrupt", "Failed to make temporary DLL", "Old CIN version", "Drag socket not found", "Failed to load drop-object", "Failed to register OLE object", "Failed to release OLE object", "Format specifier type mismatch", "Unknown format specifier", "Too few format specifiers", "Too many format specifiers", "Scan failed", "Newer CIN version", "Error converting to variant", "Runtime menu error", "Password tampered", "Variant attribute not found", "Incompatible variant data type", "Event data is not available", "Event Store is not present", "Occurrence is not found", "Event Queue is not created", "Event info is not available", "Refnum passed is NULL", "Error retrieving Class GUID", "Error retrieving CoClass GUID", "Error retrieving TypeLib GUID.", "Bad built application magic bytes.", "Specific driver is different from the specific driver associated with the Logical Name.", "There is no session opened to the class driver.", "Max Error", "MAX - Error with config objects", "MAX - Error loading configuration", "MAX - Group not supported"]
        # "Current State"
        # "Do not delete, rename, or modify this frame.\n(this is used to capture unhandled states and typos)"
        # "Handle mistyped state name (developer tool)"
        n89 = call <vilib>:"Add State(s) to Queue__jki_lib_state_machine.vi"("State(s) in (\"\")"=w170) -> ("States Out"=w169:string)  [unwired: 14 in]
        n90 = Format Into String(format string="Software Exception: Unhandled State \"%s\"." ("message"), error in=w171, w166) -> (resulting string=w174:string, error out=w173:errorcluster)  [unwired: 1 in]
        n91 = call <vilib>:"Error Cluster From Error Code.vi"("show call chain? (False)"=TRUE, "error in (no error)"=w173, "error message (\"\")"=w174, "error code (0)"=w175) -> ("error out"=w172:errorcluster)  [unwired: 5 in]
      }
      frame "Initialize Core Data" {
        # "Do not delete, rename, or modify this frame.\n(this is used to determine panel behavior on exit)"
        # "originally closed?"
        # "exe?"
        # "If panel starts closed or is an EXE, then close it when we exit"
        n92 = call <vilib>:"Add State(s) to Queue__jki_lib_state_machine.vi"("State(s) in (\"\")"=w188) -> ("States Out"=w187:string)  [unwired: 14 in]
        n93 = property class="VI"() -> ("Front Panel.Open"=w184:bool)  [unwired: 2 in, 2 out]
        n94 = Not(x=w184) -> (.not. x?=w181:bool)
        n95 = property class="App"() -> ("App.Kind"=w183:T18)  [unwired: 2 in, 2 out]
        n96 = Equal?(x=w183, y=T18."Run Time System" ("Application:Kind")) -> (x = y?=w180:bool)
        n97 = control-ref of="Current VI Reference"() -> (w177:refnum<vi>)
        n98 = Or(x=w181, y=w180) -> (x .or. y?=w178:bool)
        n99 = Bundle By Name(cluster=w179, "Core.Current VI Reference"=w177, "Core.Close Panel on Exit?"=w178) -> (w186:T21)
      }
      frame "Error Handler" {
        # "Unhandled Error -- Display it"
        # "Handle any errors here.\nYou can also output any states to clean-up after errors occur"
        # "Clear error"
        n100 = call <vilib>:"General Error Handler.vi"("error in (no error)"=w190) -> ()  [unwired: 10 in, 5 out]
        n101 = call <vilib>:"Add State(s) to Queue__jki_lib_state_machine.vi"("State(s) in Front (\"\")"="/* Post Error States", "State(s) in (\"\")"=w194) -> ("States Out"=w193:string)  [unwired: 13 in]
      }
      frame "Exit" {
        # "Do not put any code in this frame.\n(No errors that occur here will be handled.)"
        n102 = call <vilib>:"Add State(s) to Queue__jki_lib_state_machine.vi"("State(s) in (\"\")"=w199) -> ("States Out"=w198:string)  [unwired: 14 in]
      }
      frame "---------- Data ----------" {
        # "Do not put any code in this frame.\n(It is a separator no-op. You can make a copy of this frame to create a new Data frame)"
        n103 = call <vilib>:"Add State(s) to Queue__jki_lib_state_machine.vi"("State(s) in (\"\")"=w203) -> ("States Out"=w202:string)  [unwired: 14 in]
      }
      frame "Data: Initialize" {
        w204 = T22 {"STOP queue"=refnum, "SuperGUI ref"=refnum}  # SuperGUI
        w205 = T23 {"Current VI Reference"=refnum, "Close Panel on Exit?"=FALSE}  # Core
        w207 = TRUE  # Your Boolean data
        # "Initialize the shift-register data, here.\n(data names are defined by what you wire into the bundle function)"
        n104 = call <vilib>:"Add State(s) to Queue__jki_lib_state_machine.vi"("State(s) in (\"\")"=w211) -> ("States Out"=w210:string)  [unwired: 14 in]
        n105 = Bundle("Core"=w205, "Your Boolean data"=w207, "active cams"="active cams", "SuperGUI"=w204) -> (w209:T21)  [unwired: 1 in]
      }
      frame "Data: Cleanup" {
        # "Cleanup any data and references, here.\n(this is called automatically, by the Macro: Exit)"
        n106 = Unbundle By Name(w212) -> ("Core.Current VI Reference"=w215:refnum<vi>)
        n107 = call <vilib>:"Add State(s) to Queue__jki_lib_state_machine.vi"("State(s) in (\"\")"=w217) -> ("States Out"=w216:string)  [unwired: 14 in]
        n108 = Close Reference(reference=w215, error in (no error)=w214) -> (error out=w213:errorcluster)
      }
      frame "---------- UI ----------" {
        # "Do not put any code in this frame.\n(It is a separator no-op. You can make a copy of this frame to create a new UI frame)"
        n109 = call <vilib>:"Add State(s) to Queue__jki_lib_state_machine.vi"("State(s) in (\"\")"=w221) -> ("States Out"=w220:string)  [unwired: 14 in]
      }
      frame "UI: Initialize" {
        # "Initialize the User Interface, here.\n(this is called automatically, by the Macro: Init)"
        n110 = call <vilib>:"Add State(s) to Queue__jki_lib_state_machine.vi"("State(s) in (\"\")"=w226) -> ("States Out"=w225:string)  [unwired: 14 in]
        n111 = call <userlib>:"Fit VI window to Largest Dec__ogtk.vi"("error in (no error)"=w223) -> ("error out"=w222:errorcluster)  [unwired: 5 in, 1 out]
      }
      frame "UI: Get Device Name" {
        # "Initialize the User Interface, here.\n(this is called automatically, by the Macro: Init)"
        n112 = call <vilib>:"Add State(s) to Queue__jki_lib_state_machine.vi"("State(s) in (\"\")"=w232) -> ("States Out"=w231:string)  [unwired: 14 in]
        n113 = First Call?() -> (First Call?: T/F=w229:bool)
        n114 = case shown="True" w229 {
          tunnel: w228 -> [w233 w235]
          tunnel: [w233 w234] -> w227
          frame False {
          }
          frame True {
            n115 = disable-structure "Get Device name from control for vi mode\nand command line arg for exe" shown="RUN_TIME_ENGINE==True" {
              disable-tunnel: w235 -> [w236 w238]
              disable-tunnel: [w236 w237] -> w234
              frame condition #0 (active) {
              }
              frame condition #1 {
                n116 = control-ref of="This Application"() -> (w246:refnum<vi>)
                n117 = property class="App"(reference=w246) -> ("App.Args"=w245:string[])  [unwired: 1 in, 2 out]
                n118 = Index Array(array=w245, index #1=1 ("index")) -> (element #1=w239:string)  [unwired: 2 in, 2 out]
                n119 = Empty String/Path?(string/path=w239) -> (empty?=w243:bool)
                n120 = Concatenate Strings(w239, "_GUI ") -> (w241:string)
                n121 = case shown="False" w243 {
                  tunnel: w239 -> [w247 _]
                  frame False {
                    n122 = local write "GUIdevice 1"(w247) -> ()
                  }
                  frame True {
                  }
                }
                n123 = control-ref of="This VI"() -> (w242:refnum<vi>)
                n124 = property class="VI"(reference=w242, error in=w238, "Front Panel.Title"=w241) -> (error out=w237:errorcluster)  [unwired: 1 out]
              }
            }
          }
        }
      }
      frame "UI: Start SuperGUI" {
        # "create stop queue for supergui and its clones"
        # "x100 abort will be dependent on caller VI\nx80 abort will be independent of caller vi, this will abort vi when labview is closed."
        # "Start SuperGUI asynchronous way"
        n125 = vi-ref "GUI_Master_subvi_reentrant_queues.vi"() -> (w250:refnum<vi>)
        n126 = property class="VI"(reference=w250) -> ("Path"=w249:path)  [unwired: 1 in, 2 out]
        n127 = control-ref of="This Application"() -> (w256:refnum<vi>)
        n128 = Open VI Reference(type specifier VI Refnum (for type only)=refnum<vi> refnum, vi path=w249, options=256) -> (vi reference=w265:refnum<vi>, error out=w264:errorcluster)  [unwired: 3 in]
        n129 = Create User Event(user event datatype=T19 {"EventEnum"=enum."new data", "Device name"="Device name"} ("New Event"), error in=w252) -> (user event=w253:refnum<user-event>, error out=w259:errorcluster)
        "tcp data event" <- w253
        n130 = control-ref of="This VI"() -> (w255:refnum<vi>)
        n131 = register-events(w253) -> ()  [unwired: 2 in, 2 out]
        n132 = call "supergui create stop queue.vi"() -> ("STOP Queue out"=w261:refnum<queue>)  [unwired: 11 in]
        n133 = Current VI's Menubar() -> (w254:refnum<k9>)
        n134 = call-by-ref "Start Asynchronous Call"(reference=w265, error in=w264, "STOP Queue in"=w261, "This Application"=w256, 8:"error in (no error)"=w259, "tcp data event"=w253, "Caller menu reference"=w254, "Caller VI ref"=w255) -> (reference out=w248:refnum<vi>, error out=w251:errorcluster)  [unwired: 5 in, 1 out]
        n135 = Bundle By Name(cluster=w258, "SuperGUI.SuperGUI ref"=w248, "SuperGUI.STOP queue"=w261) -> (w257:T21)
        n136 = call <vilib>:"Add State(s) to Queue__jki_lib_state_machine.vi"("State(s) in (\"\")"=w267) -> ("States Out"=w266:string)  [unwired: 14 in]
      }
      frame "UI: Stop SuperGUI" {
        # "Stop Supergui Clone and wait until it exit properly"
        n137 = call <vilib>:"Add State(s) to Queue__jki_lib_state_machine.vi"("State(s) in (\"\")"=w275) -> ("States Out"=w274:string)  [unwired: 14 in]
        n138 = Unbundle By Name(w270) -> ("SuperGUI.SuperGUI ref"=w272:refnum<vi>, "SuperGUI.STOP queue"=w271:refnum<queue>)
        n139 = Release Queue(queue=w271, error in (no error)=w269) -> (error out=w273:errorcluster)  [unwired: 1 in, 2 out]
        n140 = call-by-ref "Wait On Asynchronous Call"(reference=w272, error in=w273) -> ("error out"=w268:errorcluster)  [unwired: 11 in, 2 out]
      }
      frame "UI: Cursor Set" {
        # "Argument"
        # "Set and Unset Cursor Busy.\n(Usage: \"UI: Cursor Set >> Busy|Idle\")"
        n141 = call <vilib>:"Add State(s) to Queue__jki_lib_state_machine.vi"("State(s) in (\"\")"=w281) -> ("States Out"=w280:string)  [unwired: 14 in]
        n142 = case shown="\"Idle\", Default" w276 {
          tunnel: w278 -> [w283 w285]
          tunnel: [w282 w284] -> w277
          frame "Idle", Default {
            n143 = call <vilib>:"Unset Busy.vi"("error in (no error)"=w283) -> ("error out"=w282:errorcluster)  [unwired: 10 in]
          }
          frame "Busy" {
            n144 = call <vilib>:"Set Busy.vi"("error in (no error)"=w285) -> ("error out"=w284:errorcluster)  [unwired: 9 in, 1 out]
          }
        }
      }
      frame "UI: Front Panel State" {
        # "Argument"
        # "Set Front Panel Open or Closed\n(Usage: \"UI: Front Panel State >> Open|Close\")"
        n145 = call <vilib>:"Add State(s) to Queue__jki_lib_state_machine.vi"("State(s) in (\"\")"=w292) -> ("States Out"=w291:string)  [unwired: 14 in]
        n146 = Unbundle By Name(w288) -> ("Core.Current VI Reference"=w287:refnum<vi>)
        n147 = case shown="\"Open\", Default" w286 {
          tunnel: w290 -> [w296 w309]
          tunnel: [w298 w310] -> w289
          tunnel: w287 -> [w297 w307]
          frame "Open", Default {
            n148 = property class="VI"(reference=w297, error in=w296) -> (reference out=w294:refnum<vi>, error out=w295:errorcluster, "Front Panel.Open"=w293:bool)
            n149 = case shown="False" w293 {
              tunnel: [w301 w304] -> w298
              tunnel: w295 -> [w300 w304]
              tunnel: w294 -> [w299 _]
              frame False {
                n150 = invoke class="VI" method="FP.Open"(reference=w299, error in=w300, "Activate"=TRUE, "State"=T20."Standard") -> (error out=w301:errorcluster)  [unwired: 1 in, 4 out]
              }
              frame True {
              }
            }
          }
          frame "Close" {
            n151 = property class="VI"(reference=w307, error in=w309) -> (reference out=w306:refnum<vi>, error out=w308:errorcluster, "Front Panel.Open"=w305:bool)
            n152 = case shown="True" w305 {
              tunnel: [w311 w314] -> w310
              tunnel: w308 -> [w311 w313]
              tunnel: w306 -> [_ w312]
              frame False {
              }
              frame True {
                n153 = invoke class="VI" method="FP.Close"(reference=w312, error in=w313) -> (error out=w314:errorcluster)  [unwired: 1 in, 2 out]
              }
            }
          }
        }
      }
      frame "---------- Macro ----------" {
        # "Do not put any code in this frame.\n(It is a separator no-op. You can make a copy of this frame to create a new Macro frame)"
        n154 = call <vilib>:"Add State(s) to Queue__jki_lib_state_machine.vi"("State(s) in (\"\")"=w318) -> ("States Out"=w317:string)  [unwired: 14 in]
      }
      frame "Macro: Initialize" {
        # "Initialization Macro\n(This is called once, when the VI starts)"
        n155 = call <vilib>:"Add State(s) to Queue__jki_lib_state_machine.vi"("State(s) in Front (\"\")"="Data: Initialize\nInitialize Core Data\nUI: Initialize\nUI: Get Device Name\nUI: Start SuperGUI\nUI: Front Panel State >> Open", "State(s) in (\"\")"=w323) -> ("States Out"=w322:string)  [unwired: 13 in]
      }
      frame "Macro: Exit" {
        # "Exit Macro\n(This is called once, when the VI exits)"
        n156 = Unbundle By Name(w331) -> ("Core.Close Panel on Exit?"=w330:bool)
        n157 = Select(t="UI: Front Panel State >> Close", s=w330, f="") -> (s? t:f=w327:string)
        n158 = call <vilib>:"Add State(s) to Queue__jki_lib_state_machine.vi"("State(s) in Front (\"\")"="UI: Stop SuperGUI" ("State(s) in Front (\"\")"), "State(s) in (\"\")"=w327, "State(s) at Back (\"\")"="Data: Cleanup\nExit") -> ("States Out"=w325:string)  [unwired: 12 in]
        n159 = call <vilib>:"Add State(s) to Queue__jki_lib_state_machine.vi"("State(s) in Front (\"\")"=w325, "State(s) in (\"\")"=w334) -> ("States Out"=w333:string)  [unwired: 13 in]
      }
      frame "---------- New Category ----------" {
        # "Template Separator\n(You can make a copy of, or modify, this frame)"
        n160 = call <vilib>:"Add State(s) to Queue__jki_lib_state_machine.vi"("State(s) in (\"\")"=w338) -> ("States Out"=w337:string)  [unwired: 14 in]
      }
      frame "New Category: 1" {
        # "Your code here.\n(You can make a copy of, or modify, this frame)"
        n161 = call <vilib>:"Add State(s) to Queue__jki_lib_state_machine.vi"("State(s) in (\"\")"=w342) -> ("States Out"=w341:string)  [unwired: 14 in]
      }
      frame "New Category: 2" {
        # "Your code here.\n(You can make a copy of, or modify, this frame)"
        n162 = call <vilib>:"Add State(s) to Queue__jki_lib_state_machine.vi"("State(s) in (\"\")"=w346) -> ("States Out"=w345:string)  [unwired: 14 in]
      }
    }
  }
